vi "Router - Connect.vi"(8 "error in (no error)":errorcluster, 11 "Router Data In":T1) -> (0 "error out":errorcluster, 3 "Router Data Out":T1)   [LabVIEW 2016, in "PXImc Router.lvlib"]
uses:
  PXImc Router.lvlib
  Controls/Router - Configuration.ctl
  Controls/Router/Node Block R-W Properties.ctl
  Controls/Router/Block Properties.ctl
  Controls/Router/Router - PXImc Properties.ctl
  Controls/Router/Router - PXImc Card Properties.ctl
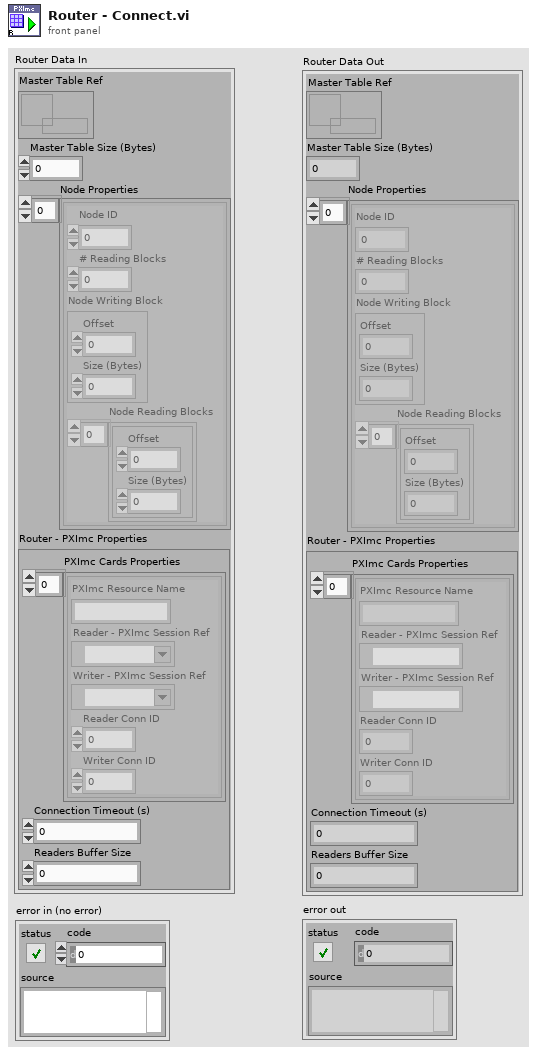
[diagram p1: front panel]
types:
  T1 = typedef "PXImc Router.lvlib/Router - Configuration.ctl" = cluster{"Master Table Ref":refnum<data-value>, "Master Table Size (Bytes)":u32, "Node Properties":T2[], "Router - PXImc Properties":T4}
  T2 = typedef "PXImc Router.lvlib/Node Block R-W Properties.ctl" = cluster{"Node ID":u32, "# Reading Blocks":u32, "Node Writing Block":T3, "Node Reading Blocks":T3[]}
  T3 = typedef "PXImc Router.lvlib/Block Properties.ctl" = cluster{"Offset":u32, "Size (Bytes)":u32}
  T4 = typedef "PXImc Router.lvlib/Router - PXImc Properties.ctl" = cluster{"PXImc Cards Properties":T5[], "Connection Timeout (s)":dbl, "Readers Buffer Size":u64}
  T5 = typedef "PXImc Router.lvlib/Router - PXImc Card Properties.ctl" = cluster{"PXImc Resource Name":string, "Reader - PXImc Session Ref":refnum<k21>, "Writer - PXImc Session Ref":refnum<k21>, "Reader Conn ID":u16, "Writer Conn ID":u16}
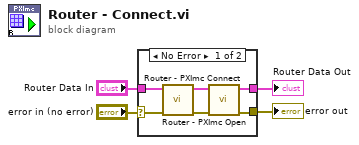
[diagram p0: block diagram]
diagram:
  n1 = case shown="No Error" "error in (no error)" {
    selector: "error in (no error)" -> [w9 w12]
    tunnel: [w6 w12] -> w3
    tunnel: "Router Data In" -> [w10 w11]
    tunnel: [w5 w11] -> w1
    frame No Error {
      n2 = call "Router - PXImc Open.vi"("error in (no error)"=w9, "Router Data In"=w10) -> ("error out"=w8:errorcluster, "Router Data Out"=w7:T1)  [unwired: 8 in]
      n3 = call "Router - PXImc Connect.vi"("error in (no error)"=w8, "Router Data In"=w7) -> ("error out"=w6:errorcluster, "Router Data Out"=w5:T1)  [unwired: 8 in]
    }
    frame Error {
    }
  }
  "error out" <- w3
  "Router Data Out" <- w1
